vi "Bootstrap.vi"(7 "Open FP":bool, 8 "error in (no error)":errorcluster, 9 "Name":string, 10 "Controller.lvclass":refnum<class "Controller.lvclass">, 11 "vi path":path) -> (0 "error out":errorcluster, 2 "Is Running?":bool, 3 "Module out":refnum<class "Module.lvclass">)   [LabVIEW 2020, in "Module.lvclass"]
uses:
  Module.lvclass
  Controller/Controller.lvclass
  Controller/Controller.lvclass/Controller.ctl
  controls/Request.ctl
  Module.lvclass/Module.ctl
  Controller/Get E-Stop Event.vi
  Controller/Get Logging.vi
  Controller/Get Trunk.vi
  Controller/Get Module response.vi
  Logging/Logging.lvclass
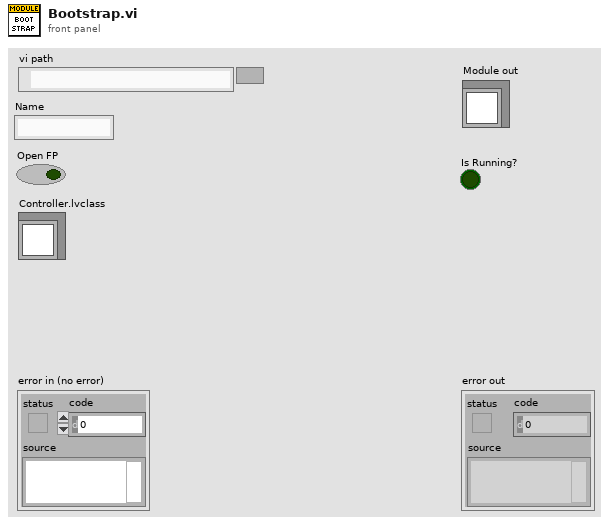
[diagram p1: front panel]
types:
  T1 = enum32{"Invalid", "Standard", "Closed", "Hidden", "Minimized", "Maximized"}
  T2 = typedef "Request.ctl" = cluster{"Method":string, "Params":variant}
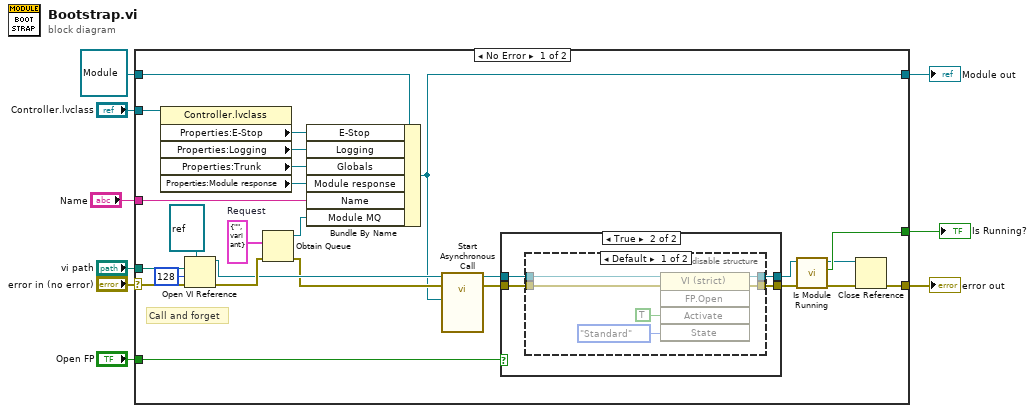
[diagram p0: block diagram]
diagram:
  n1 = case shown="No Error" "error in (no error)" {
    selector: "error in (no error)" -> [w32 w51]
    tunnel: [w11 w51] -> w8
    tunnel: [w16 w50] -> w6
    tunnel: refnum<class "Module.lvclass"> refnum ("Module in") -> [w35 w50]
    tunnel: "Controller.lvclass" -> [w34 _]
    tunnel: "Open FP" -> [w28 _]
    tunnel: [w29 _] -> w3
    tunnel: "vi path" -> [w31 _]
    tunnel: "Name" -> [w23 _]
    frame No Error {
      w20 = T2 {"Method"="", "Params"=variant}  # Request
      # "Call and forget"
      n2 = property class="Controller.lvclass"(reference=w34) -> ("Properties:E-Stop"=w22:refnum<user-event>, "Properties:Logging"=w27:refnum<class "Logging.lvclass">, "Properties:Trunk"=w26:refnum<data-value>, "Properties:Module response"=w21:refnum<user-event>)  [unwired: 1 in, 2 out]
      n3 = Open VI Reference(type specifier VI Refnum (for type only)=refnum<vi> refnum, vi path=w31, options=128, error in (no error)=w32) -> (vi reference=w19:refnum<vi>, error out=w24:errorcluster)  [unwired: 2 in]
      n4 = Obtain Queue(element data type=w20, error in (no error)=w24) -> (queue out=w25:refnum<queue>, error out=w18:errorcluster)  [unwired: 3 in, 1 out]
      n5 = Bundle By Name(cluster=w35, "E-Stop"=w22, "Logging"=w27, "Globals"=w26, "Module response"=w21, "Name"=w23, "Module MQ"=w25) -> (w16:refnum<class "Module.lvclass">)
      n6 = call-by-ref "Start Asynchronous Call"(reference=w19, error in=w18, "Module in"=w16) -> (reference out=w14:refnum<vi>, error out=w15:errorcluster)  [unwired: 11 in]
      n7 = case shown="True" w28 {
        tunnel: w15 -> [w37 w41]
        tunnel: w14 -> [w36 w40]
        tunnel: [w37 w39] -> w30
        tunnel: [w36 w38] -> w13
        frame False {
        }
        frame True {
          n8 = disable-structure shown="Default" {
            disable-tunnel: w41 -> [w47 w49]
            disable-tunnel: w40 -> [w46 w48]
            disable-tunnel: [w43 w49] -> w39
            disable-tunnel: [w42 w48] -> w38
            frame condition #0 {
              n9 = invoke class="VI (strict)" method="FP.Open"(reference=w46, error in=w47, "Activate"=TRUE ("Activate?"), "State"=T1."Standard") -> (reference out=w42:refnum<vi>, error out=w43:errorcluster)  [unwired: 1 in, 3 out]
            }
            frame condition #1 (active) {
            }
          }
        }
      }
      n10 = call "Is Module Running.vi"("error in (no error)"=w30, "VI reference in"=w13) -> ("error out"=w12:errorcluster, "Is Running?"=w29:bool, "VI reference out"=w10:refnum<vi>)  [unwired: 6 in, 1 out]
      n11 = Close Reference(reference=w10, error in (no error)=w12) -> (error out=w11:errorcluster)
    }
    frame Error {
    }
  }
  "error out" <- w8
  "Module out" <- w6
  "Is Running?" <- w3
